vi "Convert_TDMS_To_CSV.vi"() -> ()   [LabVIEW 2024]
uses:
  <vilib>/Utility/file.llb/Write Delimited Spreadsheet (string).vi
panel:
  out "Total Columns":i32
  out "Total Rows":i32
  out "Processing conversion…":u8(slide) scale=0.0..100.0
  out "Data":string[][](table)
  out "Group Name":string
  out "TDMS File Path":path
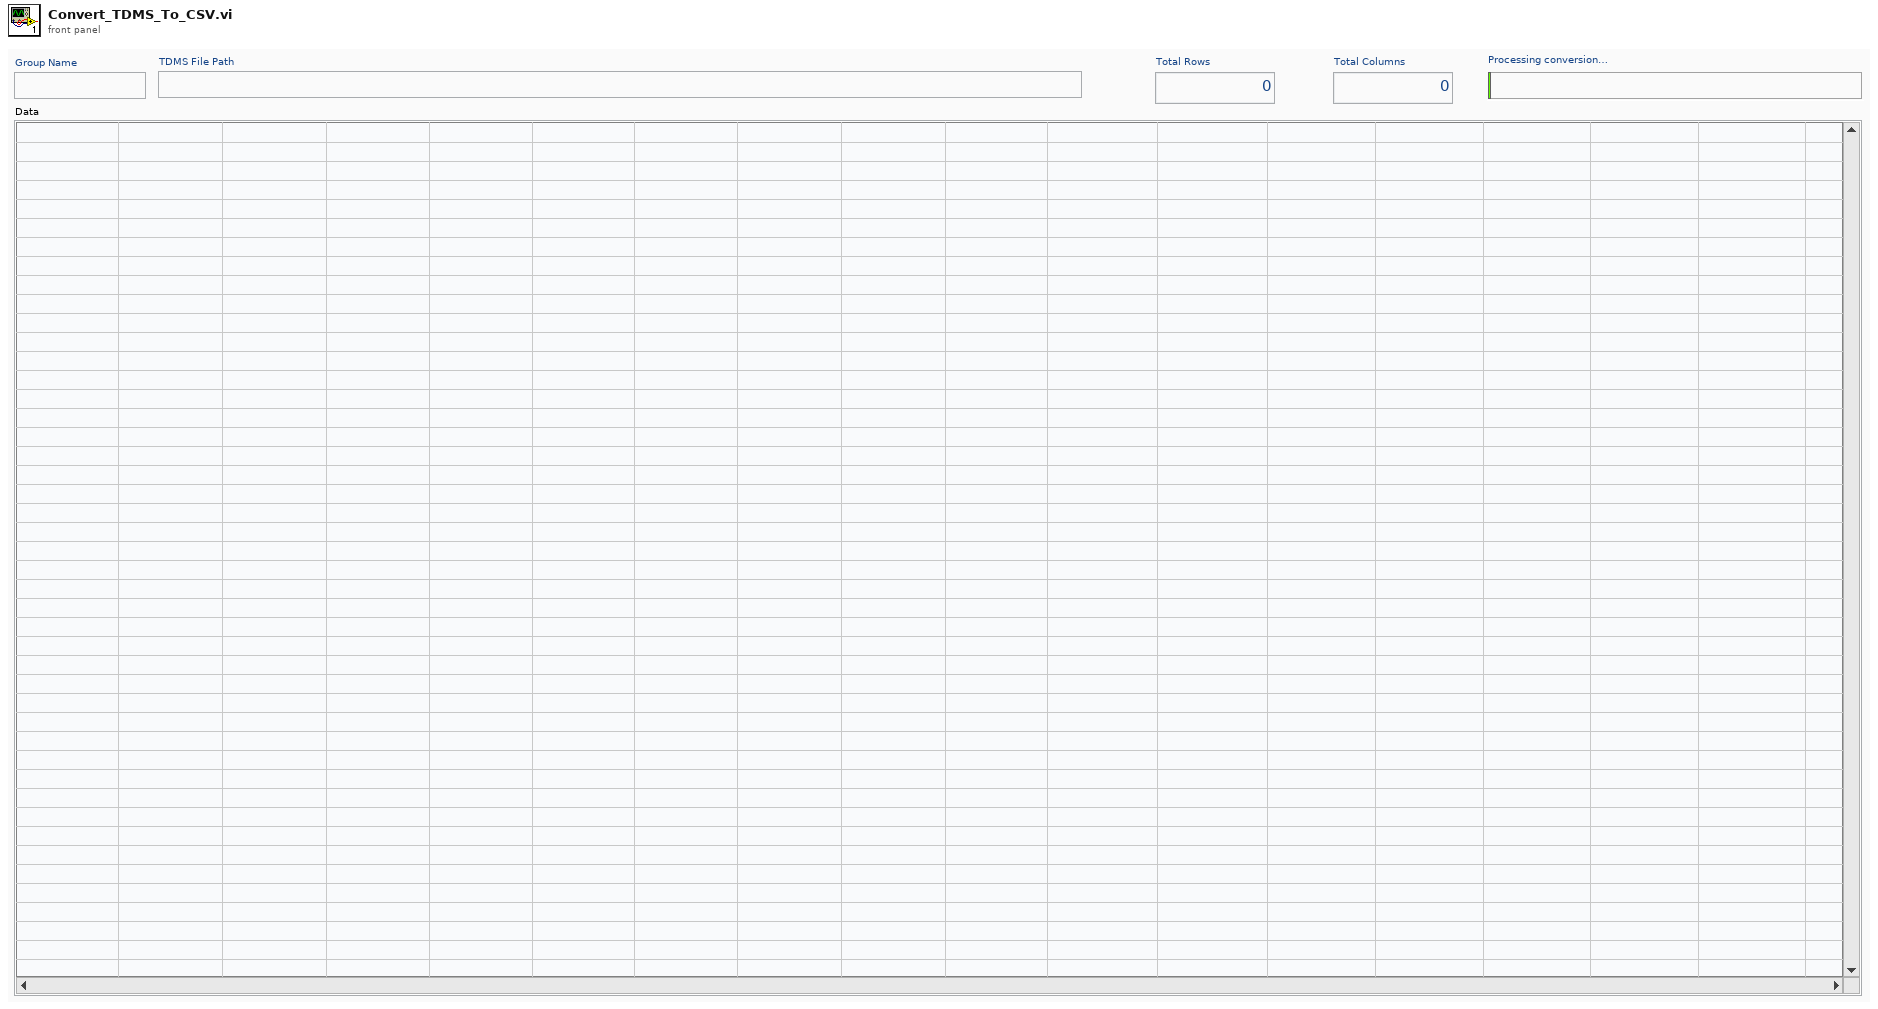
[diagram p1: front panel]
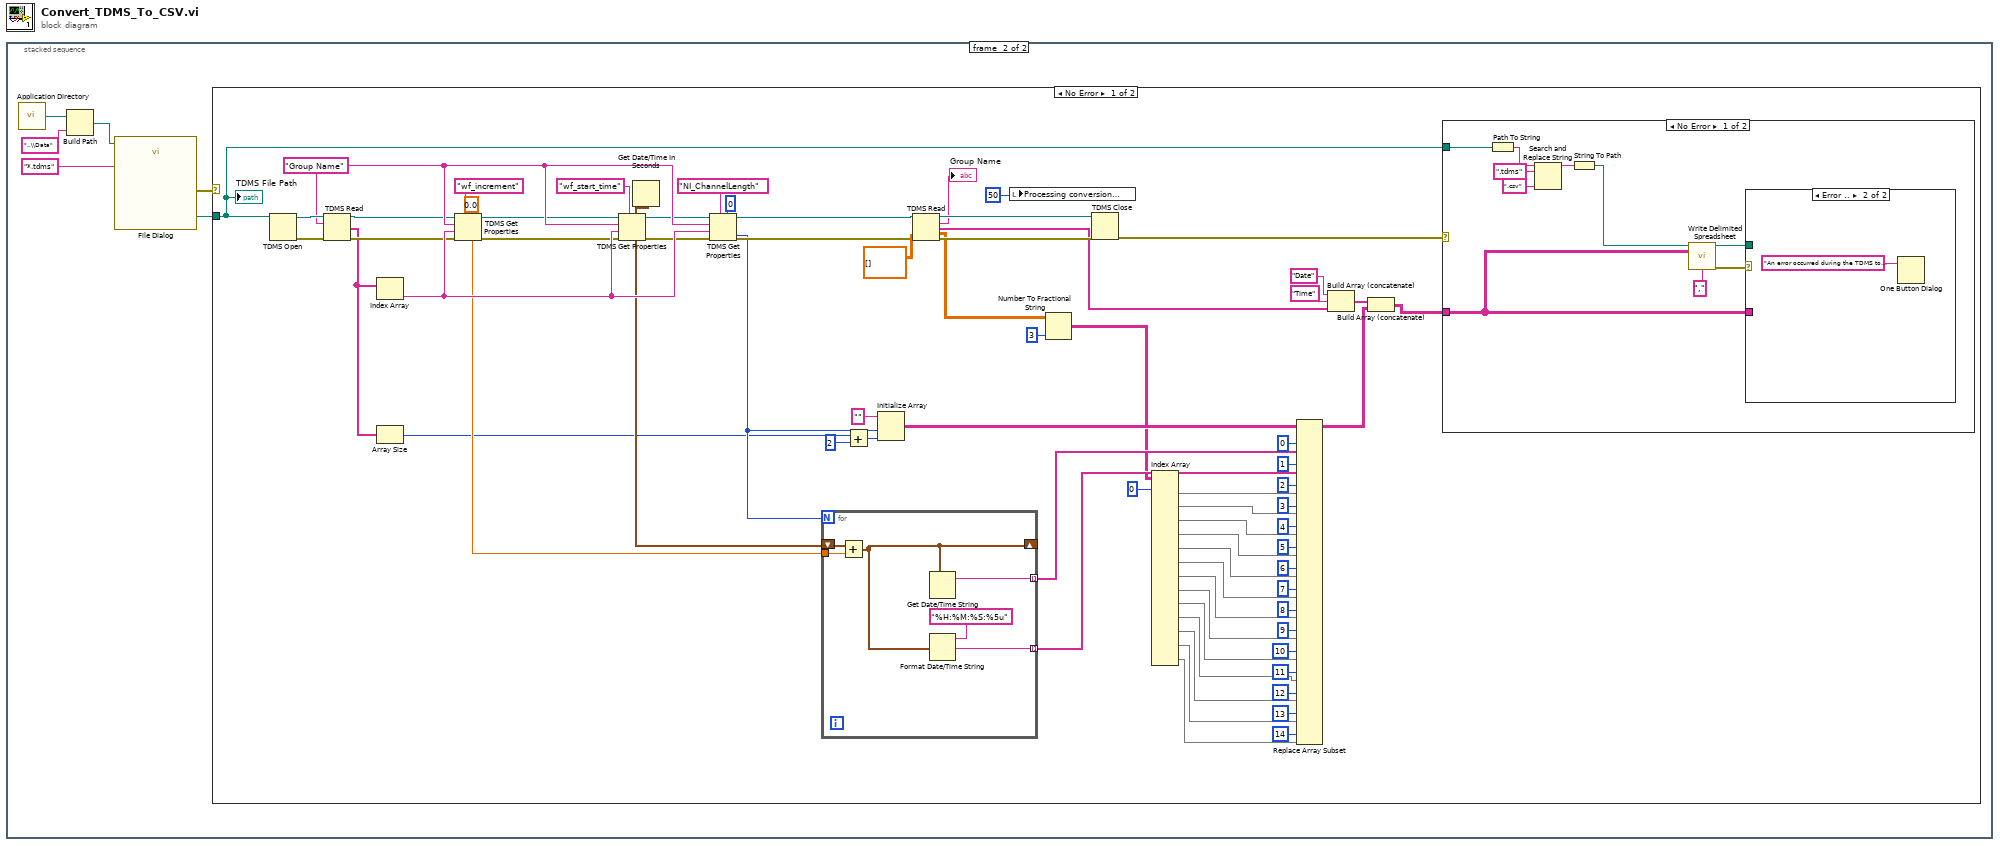
[diagram p0: block diagram]
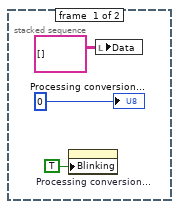
[diagram p2: hidden frame]
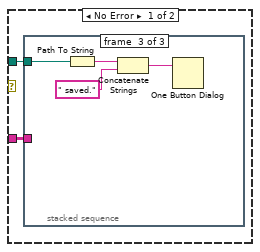
[diagram p3: hidden frame]
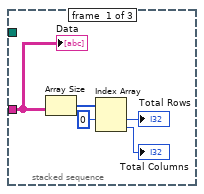
[diagram p4: hidden frame]
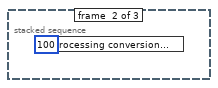
[diagram p5: hidden frame]
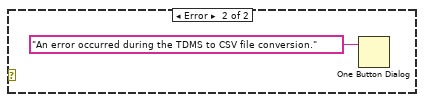
[diagram p6: hidden frame]
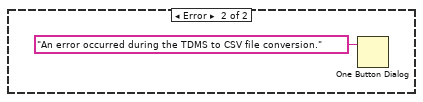
[diagram p7: hidden frame]
diagram:
  n1 = stacked-sequence {
    frame #0 {
      n2 = property on="Processing conversion…" class="Slide (strict)"("Blinking"=TRUE) -> ()  [unwired: 2 in, 2 out]
      n3 = local write "Data"(string[][] [] ("Data")) -> ()
      "Processing conversion…" <- u8 0 ("Progress Bar")
    }
    frame #1 {
      n4 = call <vilib>:"Application Directory.vi"() -> ("Application Directory"=w6:path)
      n5 = Build Path(base path=w6, name or relative path="..\\Data") -> (appended path=w4:path)
      n6 = call "File Dialog"("start path"=w4, "pattern (all files)"="*.tdms") -> ("selected path"=w9:path, "error out"=w7:errorcluster)  [unwired: 10 in, 2 out]
      n7 = case shown="No Error" w7 {
        tunnel: w9 -> [w75 _]
        frame No Error {
          w65 = "Group Name" ("group name in")
          n8 = TDMS Open(11:w75) -> (0:w73:errorcluster, 3:w67:refnum<k34>)  [unwired: 6 in]
          n9 = TDMS Read(0:w67, 5:w65, 11:w73) -> (4:w59:refnum<k34>, 8:w48:string[], 15:w58:errorcluster)  [unwired: 5 in, 3 out]
          n10 = Index Array(array=w48) -> (element=w64:string)  [unwired: 1 in]
          n11 = Array Size(array=w48) -> (size(s)=w47:i32)
          n12 = TDMS Get Properties(5:0.0, 7:"wf_increment" ("property name"), 8:w58, 9:w64, 10:w65, 11:w59) -> (0:w56:errorcluster, 3:w57:refnum<k34>, 4:w63:dbl)  [unwired: 3 out]
          n13 = Get Date/Time In Seconds() -> (seconds since 1Jan1904=w71:timestamp)
          n14 = TDMS Get Properties(5:w71, 7:"wf_start_time" ("property name"), 8:w56, 9:w64, 10:w65, 11:w57) -> (0:w54:errorcluster, 3:w55:refnum<k34>, 4:w62:timestamp)  [unwired: 3 out]
          n15 = TDMS Get Properties(5:0, 7:"NI_ChannelLength", 8:w54, 9:w64, 10:w65, 11:w55) -> (0:w60:errorcluster, 3:w61:refnum<k34>, 4:w49:i32)  [unwired: 3 out]
          n16 = for {
            N: w49 -> [_]
            tunnel: w63 -> [w89]
            shift-right: [w86] -> _
            shift-left: w62 -> [w88]
            tunnel: [w87] -> w42 mode=indexing
            tunnel: [w84] -> w40 mode=indexing
            n17 = Add(x=w88, y=w89) -> (x+y=w86:timestamp)
            n18 = Get Date/Time String(seconds (now)=w86) -> (date string=w87:string)  [unwired: 2 in, 1 out]
            n19 = Format Date/Time String(time format string (%c)="%H:%M:%S:%5u", seconds (now)=w86) -> (date/time string=w84:string)  [unwired: 1 in]
          }
          n20 = Add(x=w47, y=2) -> (x+y=w45:i32)
          n21 = Initialize Array("", w49, w45) -> (w44:string[][])
          n22 = TDMS Read(0:w61, 11:w60, 12:dbl[][] []) -> (4:w83:refnum<k34>, 6:→"Group Name":string, 8:w79:string[], 10:w13:dbl[][], 15:w82:errorcluster)  [unwired: 5 in, 1 out]
          n23 = local write "Processing conversion…"(u8 50 ("Progress Bar")) -> ()
          n24 = Number To Fractional String(number=w13, precision (6)=i16 3) -> (F-format string=w39:string[][])  [unwired: 2 in]
          n25 = TDMS Close(8:w82, 11:w83) -> (0:w76:errorcluster)  [unwired: 1 out]
          n26 = Index Array(array=w39, index (row) #1=0 ("disabled index (col)")) -> (element #1=w38:string[], element #2=w36:string[], element #3=w35:string[], element #4=w34:string[], element #5=w33:string[], element #6=w32:string[], element #7=w11:string[], element #8=w31:string[], element #9=w30:string[], element #10=w29:string[], element #11=w28:string[], element #12=w27:string[], element #13=w26:string[])  [unwired: 25 in]
          n27 = Replace Array Subset(array=w44, new element #1=w42, index (col) #1=0 ("disabled index (col)"), new element #2=w40, index (col) #2=1 ("index (col)"), new element #3=w38, index (col) #3=2 ("index (col)"), new element #4=w36, index (col) #4=3 ("index (col)"), new element #5=w35, index (col) #5=4 ("index (col)"), new element #6=w34, index (col) #6=5 ("index (col)"), new element #7=w33, index (col) #7=6 ("index (col)"), new element #8=w32, index (col) #8=7 ("index (col)"), new element #9=w11, index (col) #9=8 ("index (col)"), new element #10=w31, index (col) #10=9 ("index (col)"), new element #11=w30, index (col) #11=10 ("index (col)"), new element #12=w29, index (col) #12=11 ("index (col)"), new element #13=w28, index (col) #13=12 ("index (col)"), new element #14=w27, index (col) #14=13 ("index (col)"), new element #15=w26, index (col) #15=14 ("index (col)")) -> (w10:string[][])  [unwired: 15 in]
          n28 = Build Array (concatenate)("Date", "Time", w79) -> (w53:string[])
          n29 = Build Array (concatenate)(w53, w10) -> (w78:string[][])
          n30 = case shown="No Error" w76 {
            tunnel: w78 -> [w92 _]
            tunnel: w75 -> [w99 _]
            frame No Error {
              n31 = Path To String(path=w99) -> (string=w98:string)
              n32 = Search and Replace String(input string=w98, search string=".tdms", replace string=".csv" ("replace string (\"\")")) -> (result string=w95:string)  [unwired: 5 in, 3 out]
              n33 = String To Path(string=w95) -> (path=w94:path)
              n34 = call-poly <vilib>:"Write Delimited Spreadsheet.vi"("file path (dialog if empty)"=w94, "2D data"=w92, "delimiter (\\t)"="," ("delimiter (\\t)")) -> ("new file path (Not A Path if cancelled)"=w90:path, "error out"=w91:errorcluster)  [unwired: 11 in]
              n35 = case shown="Error .." w91 {
                tunnel: w92 -> [w100 _]
                tunnel: w90 -> [w101 _]
                frame No Error {
                  n36 = stacked-sequence {
                    tunnel: w101 -> [_ _ w111]
                    tunnel: w100 -> [w106 _ _]
                    frame #0 {
                      n37 = Array Size(array=w106) -> (size(s)=w105:i32[])
                      n38 = Index Array(array=w105, index #1=0 ("index")) -> (element #1=→"Total Rows":i32, element #2=→"Total Columns":i32)  [unwired: 1 in]
                      "Data" <- w106
                    }
                    frame #1 {
                      n39 = local write "Processing conversion…"(u8 100 ("Progress Bar")) -> ()
                    }
                    frame #2 {
                      n40 = Path To String(path=w111) -> (string=w110:string)
                      n41 = Concatenate Strings(w110, " saved." ("string")) -> (w109:string)
                      n42 = One Button Dialog(message=w109) -> ()  [unwired: 1 in, 1 out]
                    }
                  }
                }
                frame Error {
                  n43 = One Button Dialog(message="An error occurred during the TDMS to CSV file conversion.") -> ()  [unwired: 1 in, 1 out]
                }
              }
            }
            frame Error {
              n44 = One Button Dialog(message="An error occurred during the TDMS to CSV file conversion.") -> ()  [unwired: 1 in, 1 out]
            }
          }
          "TDMS File Path" <- w75
        }
        frame Error {
          n45 = One Button Dialog(message="An error occurred during the TDMS to CSV file conversion.") -> ()  [unwired: 1 in, 1 out]
        }
      }
    }
  }
